vi "Write Update period.vi"(8 "error in (no error)":errorcluster, 10 "Update period [µs]":u16, 11 "Speed in":refnum<class "Speed.lvclass">) -> (0 "error out":errorcluster, 3 "Speed out":refnum<class "Speed.lvclass">)   [LabVIEW 2013, in "HardwareCharacterization.lvlib" / "Speed.lvclass"]
uses:
  Speed.lvclass
  Speed.lvclass/Speed.ctl
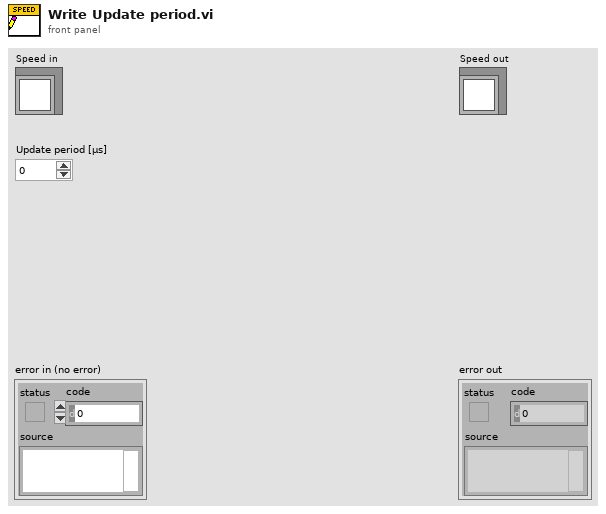
[diagram p1: front panel]
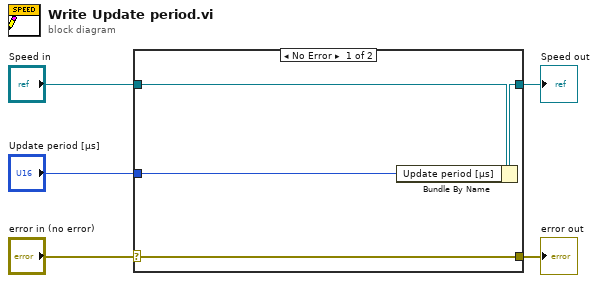
[diagram p0: block diagram]
diagram:
  n1 = case shown="No Error" "error in (no error)" {
    selector: "error in (no error)" -> [w9 w10]
    tunnel: [w9 w10] -> w4
    tunnel: [w7 w11] -> w2
    tunnel: "Speed in" -> [w8 w11]
    tunnel: "Update period [µs]" -> [w6 _]
    frame No Error {
      n2 = Bundle By Name(cluster=w8, "Update period [µs]"=w6) -> (w7:refnum<class "Speed.lvclass">)
    }
    frame Error {
    }
  }
  "error out" <- w4
  "Speed out" <- w2
